vi "Write Name Lookup Table (GUID should return Name).vi"(10 "Name Lookup Table (GUID should return Name)":variant, 11 "ServerListener in":refnum<class "ServerListener.lvclass">) -> (3 "ServerListener out":refnum<class "ServerListener.lvclass">)   [LabVIEW 2016, in "ServerListener.lvlib" / "ServerListener.lvclass"]
uses:
  ServerListener.lvclass
  ServerListener.lvclass/ServerListener.ctl
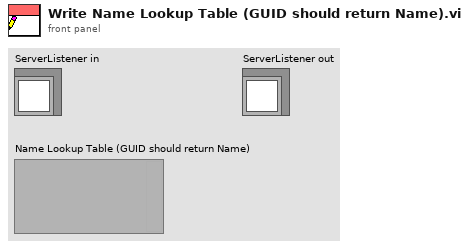
[diagram p1: front panel]
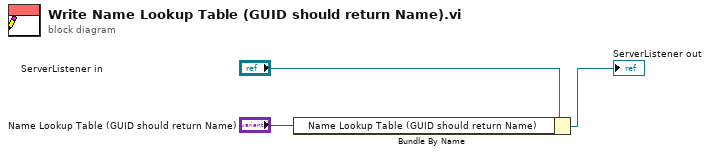
[diagram p0: block diagram]
diagram:
  n1 = Bundle By Name(cluster="ServerListener in", "Name Lookup Table (GUID should return Name)"="Name Lookup Table (GUID should return Name)") -> (→"ServerListener out":refnum<class "ServerListener.lvclass">)
